vi "Configure Hardware.vi"() -> ()   [LabVIEW 2019, in "Configure Hardware.lvlib"]
uses:
  Configure Hardware.lvlib
  support/States.ctl
  support/StateData.ctl
  Common Components/Hardware/DMM/DMM.lvclass
  Common Components/Hardware/Scope/Scope.lvclass
  Common Components/Hardware/FGEN/Function Generator.lvclass
panel:
  in  "Refresh Button":bool
  in  "DMM":i32(listbox)
  in  "Signal Generator":i32(listbox)
  in  "Scope":i32(listbox)
  # "Select Your Hardware"
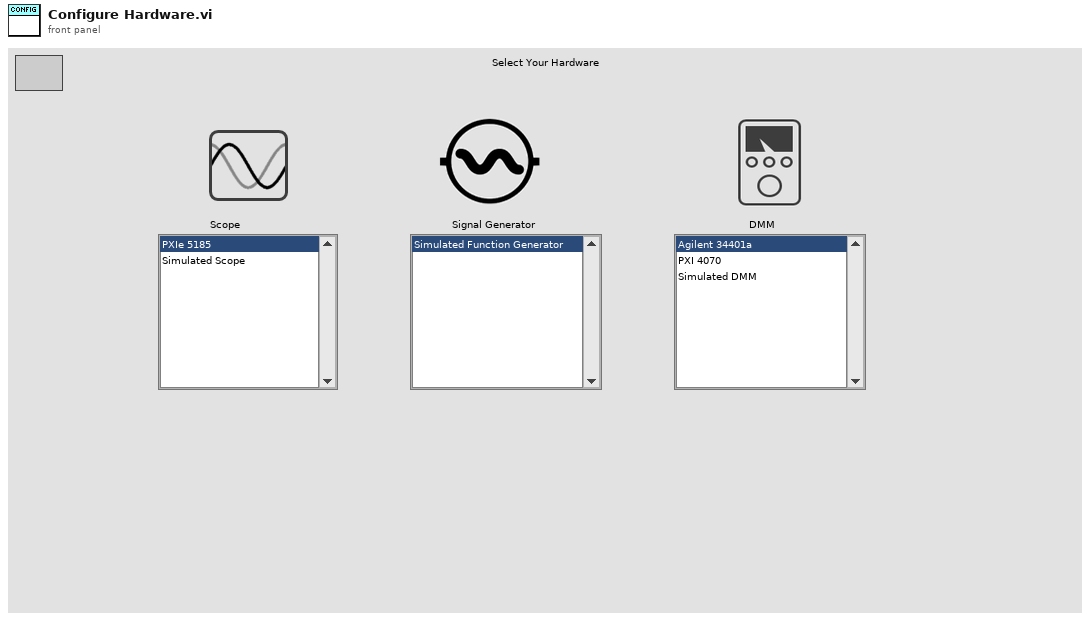
[diagram p1: front panel]
types:
  T1 = typedef "Configure Hardware.lvlib/StateData.ctl" = cluster{"DMM classes":refnum<class "DMM.lvclass">[], "Scope classes":refnum<class "Scope.lvclass">[], "FGEN classes":refnum<class "Function Generator.lvclass">[]}
  T2 = typedef "Configure Hardware.lvlib/States.ctl" = enum16{"Initialize", "Wait for Event", "Shutdown"}
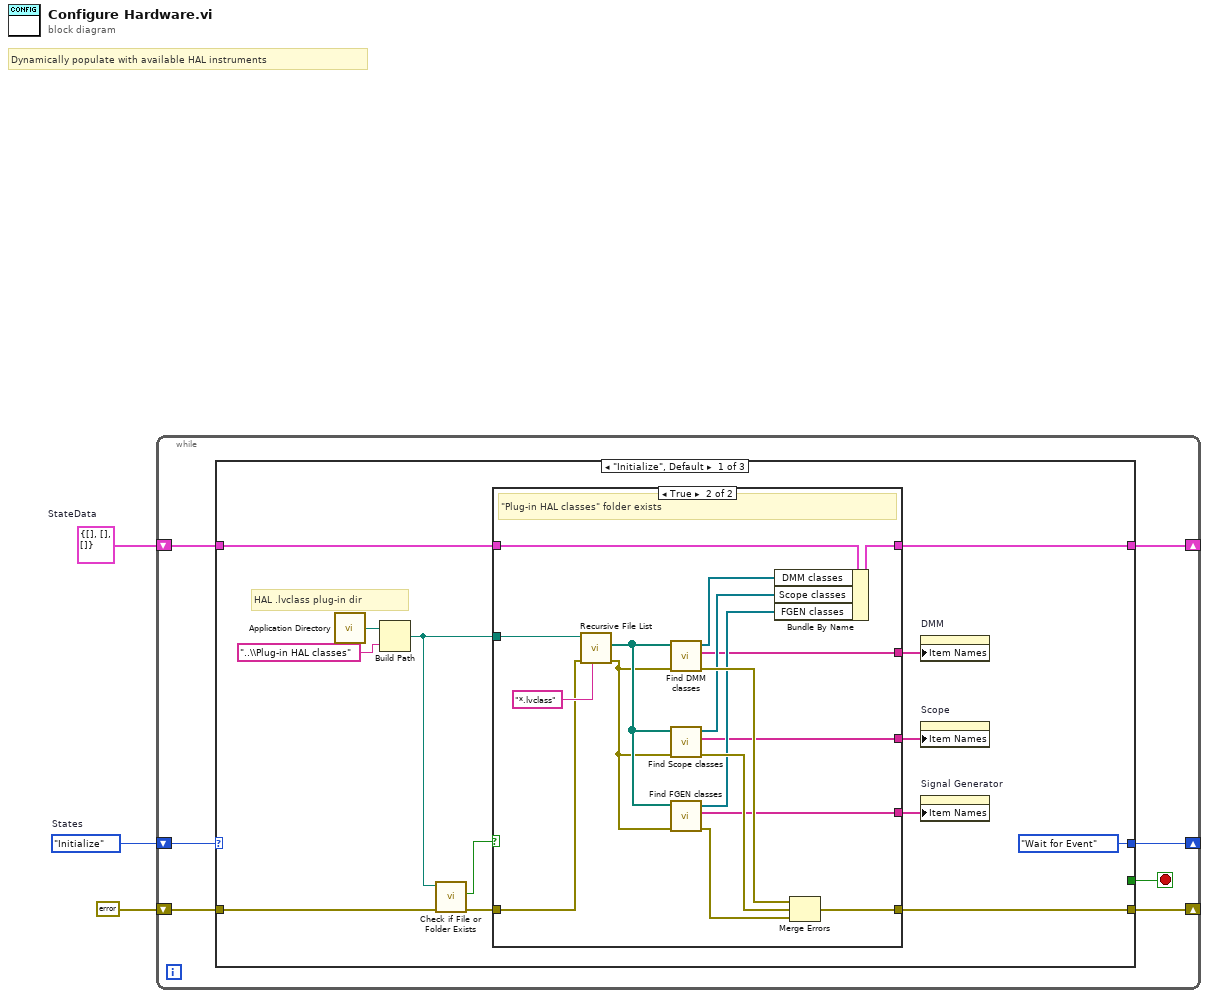
[diagram p0: block diagram]
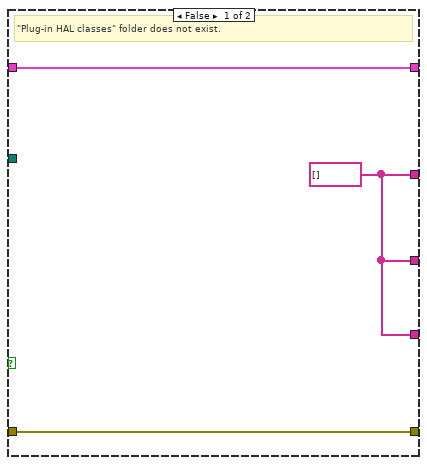
[diagram p2: hidden frame]
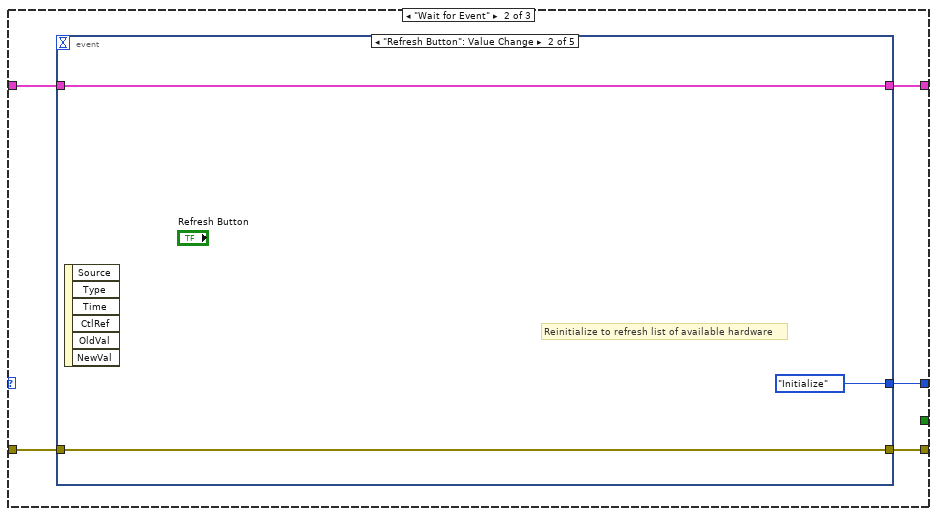
[diagram p3: hidden frame]
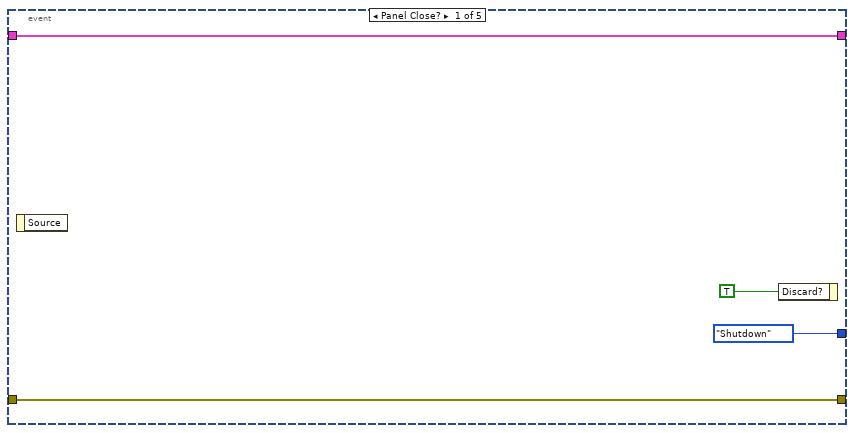
[diagram p4: hidden frame]
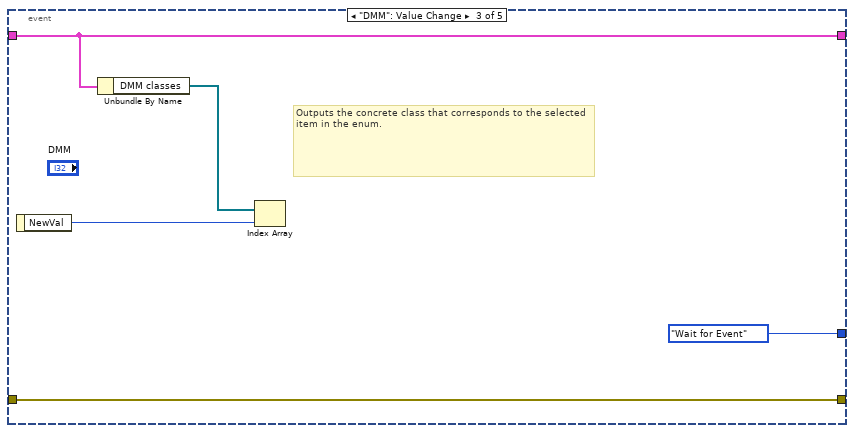
[diagram p5: hidden frame]
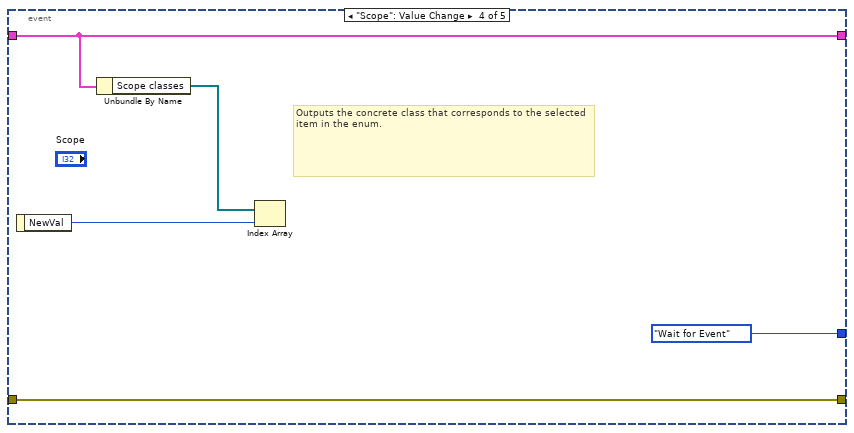
[diagram p6: hidden frame]
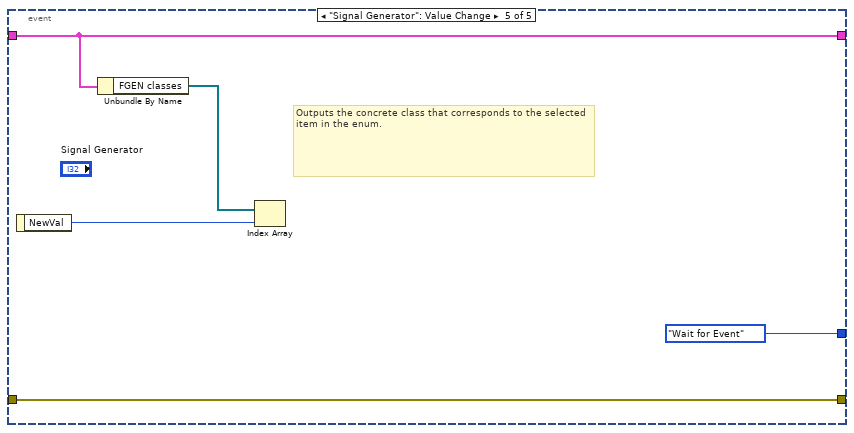
[diagram p7: hidden frame]
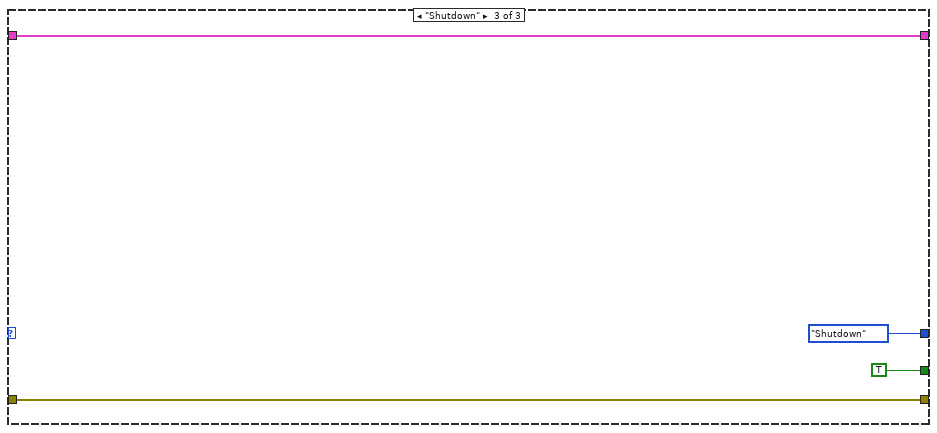
[diagram p8: hidden frame]
diagram:
  w1 = T1 {"DMM classes"=[], "Scope classes"=[], "FGEN classes"=[]}  # StateData
  w3 = States."Initialize"  # States
  # "Dynamically populate with available HAL instruments"
  n1 = while {
    shift-right: [w6] -> _
    shift-left: w3 -> [w9]
    shift-right: [w7] -> _
    shift-left: errorcluster {"status"=FALSE, "code"=0, "source"=""} ("error in (no error)") -> [w8]
    shift-right: [w4] -> _
    shift-left: w1 -> [w5]
    stop <- w10 stop-if-true
    n2 = case shown="\"Initialize\", Default" w9 {
      tunnel: [_ _ TRUE ("Discard?")] -> w10
      tunnel: w8 -> [w16 w48 w74]
      tunnel: [w22 w47 w74] -> w7
      tunnel: [States."Wait for Event" ("States") w46 States."Shutdown" ("States")] -> w6
      tunnel: w5 -> [w21 w45 w71]
      tunnel: [w20 w44 w71] -> w4
      frame "Initialize", Default {
        # "HAL .lvclass plug-in dir"
        n3 = call <vilib>:"Application Directory.vi"() -> ("Application Directory"=w19:path)
        n4 = Build Path(base path=w19, name or relative path="..\\Plug-in HAL classes") -> (appended path=w17:path)
        n5 = call <vilib>:"Check if File or Folder Exists.vi"("error in (no error)"=w16, "path"=w17) -> ("error out"=w15:errorcluster, "file or folder exists?"=w14:bool)  [unwired: 7 in, 1 out]
        n6 = case shown="True" w14 {
          tunnel: [w25 w41] -> w22
          tunnel: w21 -> [w26 w36]
          tunnel: [w26 w35] -> w20
          tunnel: w17 -> [_ w31]
          tunnel: w15 -> [w25 w30]
          tunnel: [w24 w29] -> w13
          tunnel: [w24 w28] -> w12
          tunnel: [w24 w27] -> w11
          frame False {
            w24 = string[] [] ("Class names")
            # "\"Plug-in HAL classes\" folder does not exist."
          }
          frame True {
            # "\"Plug-in HAL classes\" folder exists"
            n7 = call <vilib>:"Recursive File List.vi"("pattern"="*.lvclass", "error in (no error)"=w30, "Folder Path"=w31) -> ("error out"=w39:errorcluster, "All Files in Dir"=w40:path[])  [unwired: 4 in, 3 out]
            n8 = call "Find DMM classes.vi"("error in (no error)"=w39, "Files"=w40) -> ("error out"=w42:errorcluster, "Class names"=w27:string[], "DMM classes"=w34:refnum<class "DMM.lvclass">[])  [unwired: 7 in]
            n9 = call "Find Scope classes.vi"("error in (no error)"=w39, "Files"=w40) -> ("error out"=w38:errorcluster, "Class names"=w28:string[], "Scope classes"=w33:refnum<class "Scope.lvclass">[])  [unwired: 7 in]
            n10 = call "Find FGEN classes.vi"("error in (no error)"=w39, "Files"=w40) -> ("error out"=w37:errorcluster, "Class names"=w29:string[], "FGEN classes"=w32:refnum<class "Function Generator.lvclass">[])  [unwired: 7 in]
            n11 = Bundle By Name(cluster=w36, "DMM classes"=w34, "Scope classes"=w33, "FGEN classes"=w32) -> (w35:T1)
            n12 = Merge Errors(w42, w38, w37) -> (w41:errorcluster)
          }
        }
        n13 = property on="DMM" class="LstBox (strict)"("Item Names"=w11) -> ()  [unwired: 2 in, 2 out]
        n14 = property on="Scope" class="LstBox (strict)"("Item Names"=w12) -> ()  [unwired: 2 in, 2 out]
        n15 = property on="Signal Generator" class="LstBox (strict)"("Item Names"=w13) -> ()  [unwired: 2 in, 2 out]
      }
      frame "Wait for Event" {
        n16 = event shown="[1] \"Refresh Button\": Value Change" {
          selector: _ -> [_ _ _ _ _]
          dyn-events: _ -> [_ _ _ _ _]
          timeout: _ -> [_ _ _ _ _]
          tunnel: w48 -> [w51 w55 w60 w65 w70]
          tunnel: [w51 w55 w60 w65 w70] -> w47
          tunnel: [States."Shutdown" ("States") States."Initialize" ("States") States."Wait for Event" ("States") States."Wait for Event" ("States") States."Wait for Event" ("States")] -> w46
          tunnel: w45 -> [w49 w54 w59 w64 w69]
          tunnel: [w49 w54 w59 w64 w69] -> w44
          event Panel Close? {
            n17 = event-data() -> ()  [unwired: 1 in, 1 out]
            n18 = event-data("Discard?"=TRUE) -> ()  [unwired: 1 in, 1 out]
          }
          event "Refresh Button": Value Change {
            # "Reinitialize to refresh list of available hardware"
            n19 = event-data() -> ()  [unwired: 1 in, 6 out]
          }
          event "DMM": Value Change {
            # "Outputs the concrete class that corresponds to the selected item in the enum."
            n20 = event-data() -> ("NewVal"=w58:i32)  [unwired: 1 in]
            n21 = Unbundle By Name(w59) -> ("DMM classes"=w57:refnum<class "DMM.lvclass">[])
            n22 = Index Array(array=w57, index=w58) -> ()  [unwired: 1 out]
          }
          event "Scope": Value Change {
            # "Outputs the concrete class that corresponds to the selected item in the enum."
            n23 = event-data() -> ("NewVal"=w63:i32)  [unwired: 1 in]
            n24 = Unbundle By Name(w64) -> ("Scope classes"=w62:refnum<class "Scope.lvclass">[])
            n25 = Index Array(array=w62, index=w63) -> ()  [unwired: 1 out]
          }
          event "Signal Generator": Value Change {
            # "Outputs the concrete class that corresponds to the selected item in the enum."
            n26 = event-data() -> ("NewVal"=w68:i32)  [unwired: 1 in]
            n27 = Unbundle By Name(w69) -> ("FGEN classes"=w67:refnum<class "Function Generator.lvclass">[])
            n28 = Index Array(array=w67, index=w68) -> ()  [unwired: 1 out]
          }
        }
      }
      frame "Shutdown" {
      }
    }
  }
